vi "Read Value as JSON.vi"(8 "error in (no error)":errorcluster, 10 "Tag":string, 11 "Var Bus in":refnum<class "Omni_Bus.lvclass">) -> (0 "error out":errorcluster, 2 "JSON":string, 3 "Var Bus out":refnum<class "Omni_Bus.lvclass">)   [LabVIEW 2021, in "Omni_Bus.lvclass"]
uses:
  Omni_Bus.lvclass
  <vilib>/TSA/Abstract Data Classes/Abs_Types/Value/Abs_Value.lvclass
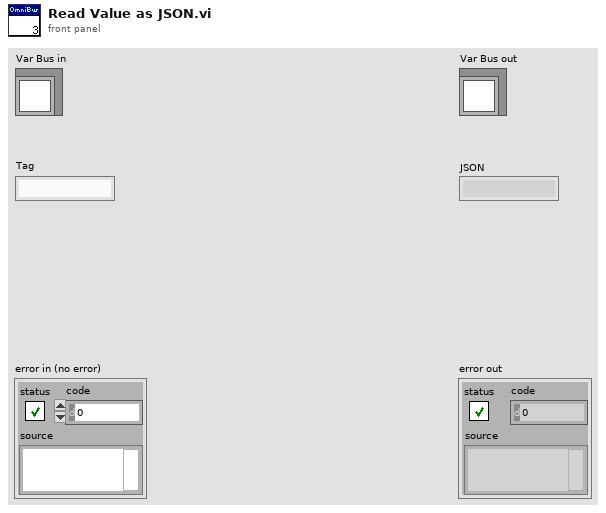
[diagram p1: front panel]
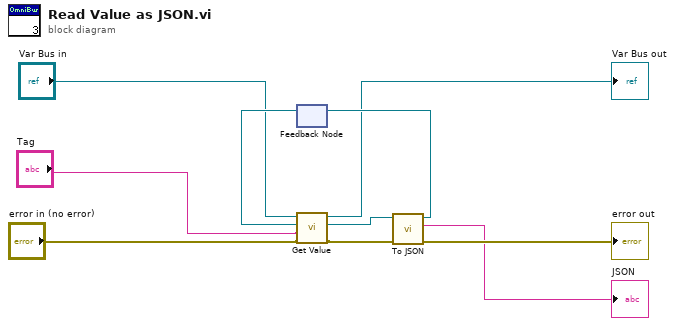
[diagram p0: block diagram]
diagram:
  n1 = feedback #1() -> (w3:refnum<class "Abs_Value.lvclass">)  [unwired: 1 in]
  n2 = call-dynamic "Get Value.vi"("error in (no error)"="error in (no error)", "Tag"="Tag", "Value Type"=w3, "Var Bus in"="Var Bus in") -> ("error out"=w7:errorcluster, "Value Out"=w6:refnum<class "Abs_Value.lvclass">, "Var Bus out"=→"Var Bus out":refnum<class "Omni_Bus.lvclass">)  [unwired: 5 in]
  n3 = call-dynamic "To JSON.vi"("error in (no error)"=w7, "Type in"=w6) -> ("error out"=→"error out":errorcluster, "JSON"=→"JSON":string, "Type out"=w8:refnum<class "Abs_Value.lvclass">)  [unwired: 7 in]
  n4 = feedback-in #1(w8) -> ()
